vi "Test Test Pass if Numeric Argument Correct.vi"(8 "error in (no error)":errorcluster, 11 "Test Case In":refnum<class "Argument Comparison Test.lvclass">) -> (0 "error out":errorcluster, 3 "Test Case Out":refnum<class "Argument Comparison Test.lvclass">)   [LabVIEW 2020, in "Argument Comparison Test.lvclass"]
uses:
  Argument Comparison Test/Argument Comparison Test.lvclass
  C:/Program Files (x86)/National Instruments/LabVIEW 2020/vi.lib/Astemes/LUnit/Test Case.lvclass
  Test Doubles/Test Interface Responsive Mock/Test Interface Responsive Mock.lvclass
  C:/git/astemes-lmock/source/Core/Mock/Mock.lvclass
  C:/git/astemes-lmock/source/Framework/Responsive Mock/Responsive Mock.lvclass
  source/Expectations/One/One.lvclass
  Expectation Test/Expectation Test.lvclass
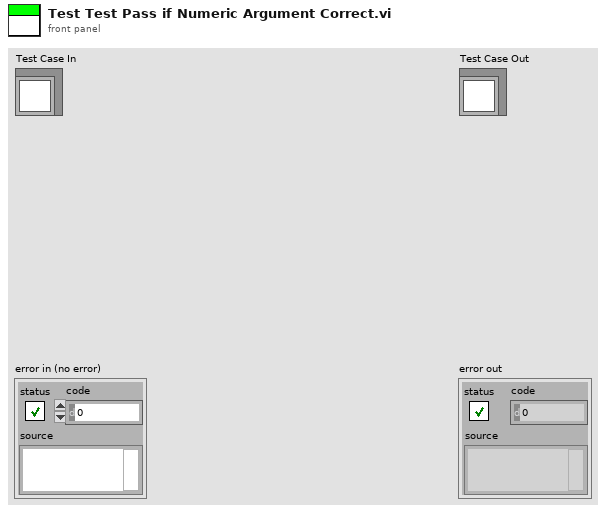
[diagram p1: front panel]
types:
  T1 = enum16{"", "Passed", "Failed", "Error", "Skipped", "Setup Error", "Broken", "Teardown Error"}
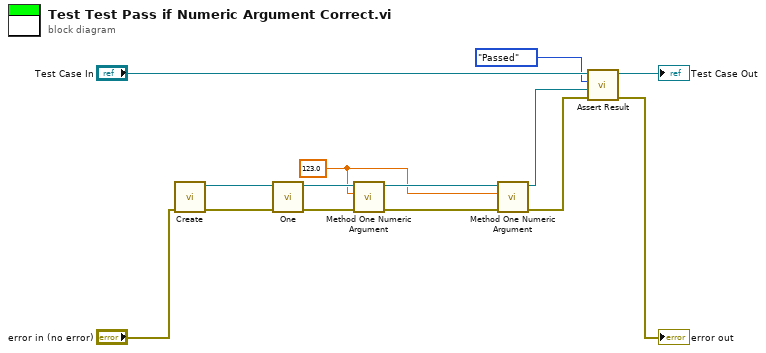
[diagram p0: block diagram]
diagram:
  w3 = 123.0 ("Numeric")
  n1 = call "Create.vi"("error in (no error)"="error in (no error)") -> ("error out"=w13:errorcluster, "Test Interface Mock Out"=w14:refnum<class "Test Interface Responsive Mock.lvclass">)  [unwired: 9 in]
  n2 = call "One.vi"("error in (no error)"=w13, "Mock in"=w14) -> ("error out"=w11:errorcluster, "Mock out"=w12:refnum<class "Test Interface Responsive Mock.lvclass">)  [unwired: 8 in]
  n3 = call-dynamic "Method One Numeric Argument.vi"("error in (no error)"=w11, "Numeric"=w3, "Test Interface Mock In"=w12) -> ("error out"=w10:errorcluster, "Test Interface Mock Out"=w4:refnum<class "Test Interface Responsive Mock.lvclass">)  [unwired: 7 in]
  n4 = call-dynamic "Method One Numeric Argument.vi"("error in (no error)"=w10, "Numeric"=w3, "Test Interface Mock In"=w4) -> ("error out"=w2:errorcluster, "Test Interface Mock Out"=w1:refnum<class "Test Interface Responsive Mock.lvclass">)  [unwired: 7 in]
  n5 = call "Assert Result.vi"("error in (no error)"=w2, "Mock"=w1, "Status"=T1."Passed", "LUnit Test Case In"="Test Case In") -> ("error out"=→"error out":errorcluster, "LUnit Test Case Out"=→"Test Case Out":refnum<class "Argument Comparison Test.lvclass">)  [unwired: 6 in]
